vi "EjSenoExcel.vi"   [LabVIEW 2020]
uses:
  <vilib>/express/express shared/transition.llb/Dynamic To Waveform Array.vi
  <vilib>/express/express signal manip/GetorSetDDTAttributes/Set DDT Attributes/SetT0.vi
  <vilib>/express/express shared/transition.llb/Waveform Array To Dynamic.vi
  <vilib>/express/express signal manip/GetorSetDDTAttributes/Set DDT Attributes/Set DDT Properties.xnode
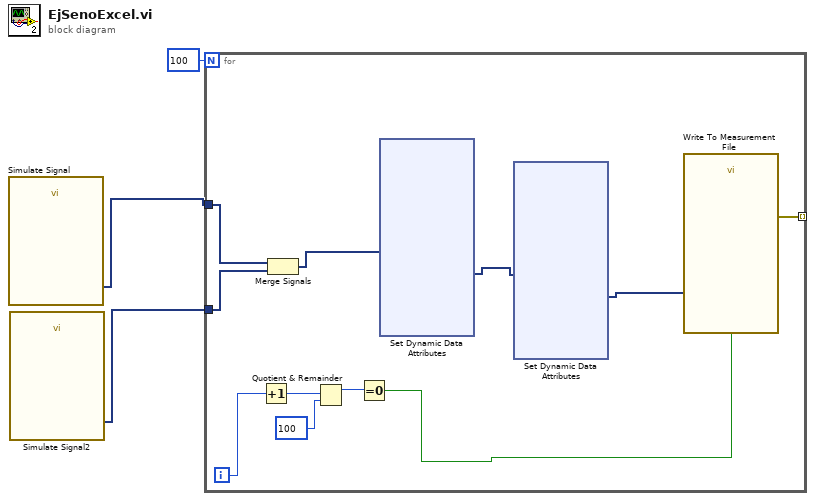
[diagram p0: block diagram]
diagram:
  n1 = call "Simulate Signal"() -> ("Sine"=w2:dynamicdata)  [unwired: 14 in, 1 out]
  n2 = call "Simulate Signal2"() -> ("Sine"=w1:dynamicdata)  [unwired: 14 in, 1 out]
  n3 = for {
    N: 100 -> [_]
    tunnel: [w14] -> _ mode=indexing
    tunnel: w2 -> [w7]
    tunnel: w1 -> [w8]
    i -> [w12]
    n4 = Increment(x=w12) -> (x+1=w13:i32)
    n5 = Merge Signals(w7, w8) -> (w4:dynamicdata)
    n6 = Quotient & Remainder(x=w13, y=100) -> (x-y*floor(x/y)=w10:i32)  [unwired: 1 out]
    n7 = Equal To 0?(x=w10) -> (x = 0?=w9:bool)
    n8 = xnode "Set Dynamic Data Attributes"("Signals In"=w4) -> ("Signals Out"=w6:dynamicdata)  [unwired: 3 in, 1 out]
    n9 = xnode "Set Dynamic Data Attributes"("Signals In"=w6) -> ("Signals Out"=w5:dynamicdata)  [unwired: 3 in, 1 out]
    n10 = call "Write To Measurement File"("Signals"=w5, "Flush? (T)"=w9) -> ("error out"=w14:errorcluster)  [unwired: 15 in, 2 out]
  }
